vi "update-raster-image.vi"(4 "detrend":bool=TRUE, 6 "current-line":i32, 7 "transpose":bool, 8 "error in (no error)":errorcluster, 9 "Master-image-in":dbl[][](array[numeric]), 10 "avg-data-row":dbl[](array[numeric]), 11 "IntensityGraph in":refnum<vi>) -> (0 "error out":errorcluster, 1 "master-image-data-out":dbl[][](array[numeric]), 3 "Intensity graph out":refnum<vi>)   [LabVIEW 2017]
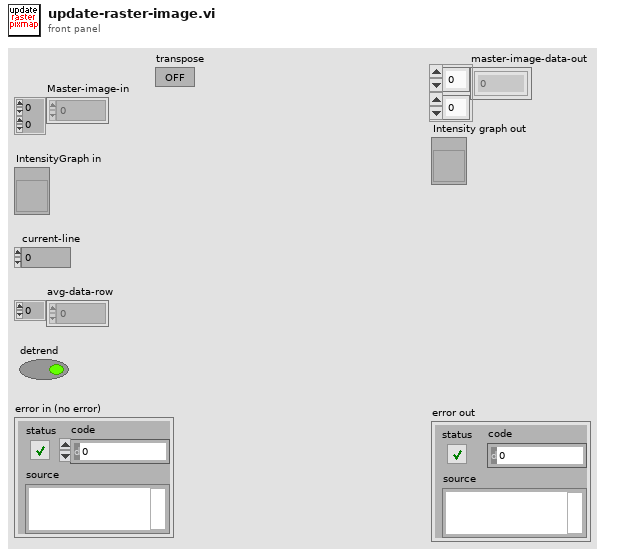
[diagram p1: front panel]
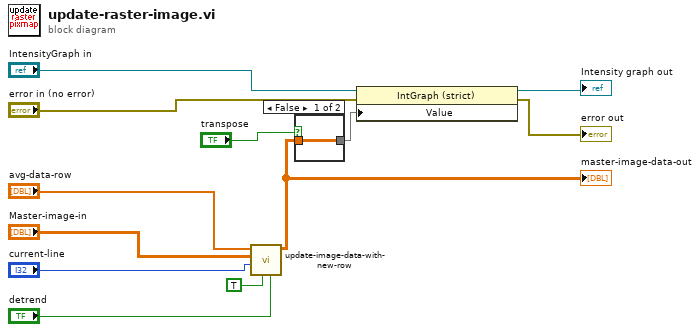
[diagram p0: block diagram]
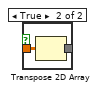
[diagram p2: hidden frame]
diagram:
  n1 = call "update-image-data-with-new-row.vi"("detrend"="detrend", "data-valid"=TRUE, "iterator"="current-line", "master-image-data-n"="Master-image-in", "avg-data-row"="avg-data-row") -> ("master-image-data-out"=w3:dbl[][])  [unwired: 6 in]
  "master-image-data-out" <- w3
  n2 = case shown="False" "transpose" {
    tunnel: w3 -> [w13 w15]
    tunnel: [w13 w14] -> w2
    frame False {
    }
    frame True {
      n3 = Transpose 2D Array(2D array=w15) -> (transposed array=w14:dbl[][])
    }
  }
  n4 = property on="Property Node" class="IntGraph (strict)"(reference="IntensityGraph in", error in="error in (no error)", "Value"=w2) -> (reference out=→"Intensity graph out":refnum<vi>, error out=→"error out":errorcluster)
